vi "Check Batch Reading Completed.vi"(3 "Profile Rsp":T1, 5 "Bufferd Profile Cnt":u32) -> (1 "Completed?":bool)   [LabVIEW 2014]
uses:
  Public/Clusters/Read Batch Profile Rsp.ctl
  Keyence LJ-V7000.lvlib
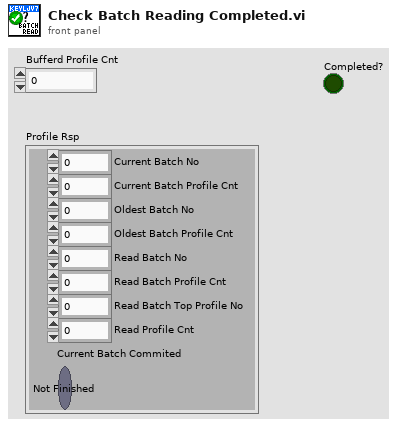
[diagram p1: front panel]
types:
  T1 = typedef "Keyence LJ-V7000.lvlib/Read Batch Profile Rsp.ctl" = cluster{"Current Batch No":u32, "Current Batch Profile Cnt":u32, "Oldest Batch No":u32, "Oldest Batch Profile Cnt":u32, "Read Batch No":u32, "Read Batch Profile Cnt":u32, "Read Batch Top Profile No":u32, "Read Profile Cnt":u8, "Current Batch Commited":bool}
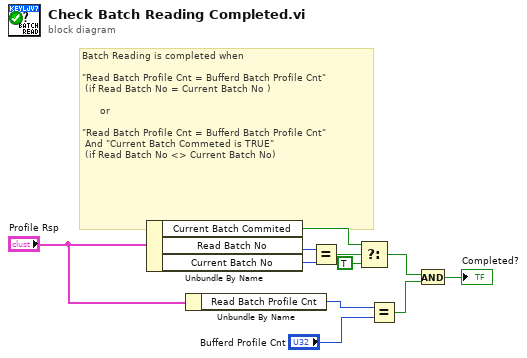
[diagram p0: block diagram]
diagram:
  # "Batch Reading is completed when\n \n\"Read Batch Profile Cnt = Bufferd Batch Profile Cnt\"\n (if Read Batch No = Current Batch No )\n\n      or\n\n\"Read Batch Profile Cnt = Bufferd Batch Profile Cnt\"\n And \"Current Batch Commeted is TRUE\"\n (if Read Batch No <> Current Batch No)"
  n1 = Unbundle By Name("Profile Rsp") -> ("Current Batch Commited"=w8:bool, "Read Batch No"=w5:u32, "Current Batch No"=w6:u32)
  n2 = Unbundle By Name("Profile Rsp") -> ("Read Batch Profile Cnt"=w11:u32)
  n3 = Equal?(x=w5, y=w6) -> (x = y?=w7:bool)
  n4 = Select(t=w8, s=w7, f=TRUE) -> (s? t:f=w3:bool)
  n5 = Equal?(x=w11, y="Bufferd Profile Cnt") -> (x = y?=w2:bool)
  n6 = And(x=w3, y=w2) -> (x .and. y?=→"Completed?":bool)
